vi "formatMsgDetails.vi"(8 "error in (no error)":errorcluster, 9 "msgTypeEnum":T1, 10 "msgCluster":T2={"msgName"="move", "msgDetails"=""}, 11 "TcpServer.lvclass":refnum<class "TcpServer.lvclass">) -> (0 "error out":errorcluster, 2 "jsonString":string, 3 "TcpServer.lvclass":refnum<class "TcpServer.lvclass">)   [LabVIEW 2018, in "TcpServer.lvclass"]
doc: "Convert the event or the telemetry message into a JSON format. You can choose if is event or telemetry with the message type enum provided. If msgName has an empty string, an error message will be created to inform other processes about this error."
uses:
  TcpServer.lvclass
  typedef/msgTypeDef.ctl
  typedef/msgTypeEnum.ctl
  <vilib>/Utility/error.llb/Error Cluster From Error Code.vi
  <vilib>/ErrorRing/Error Ring.xnode
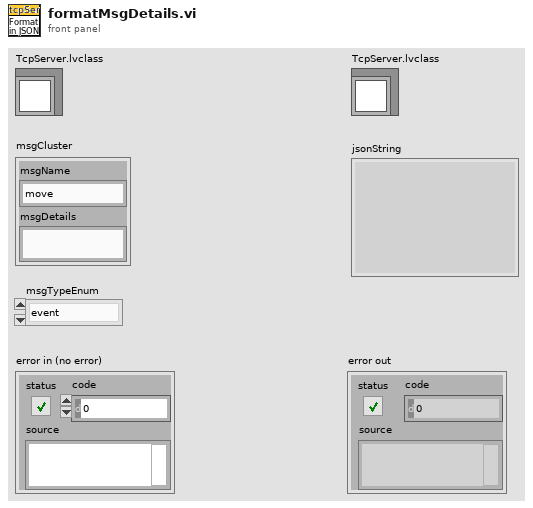
[diagram p1: front panel]
types:
  T1 = typedef "TcpServer.lvclass/msgTypeEnum.ctl" = enum16{"event", "telemetry"}
  T2 = typedef "TcpServer.lvclass/msgTypeDef.ctl" = cluster{"msgName":string, "msgDetails":string}
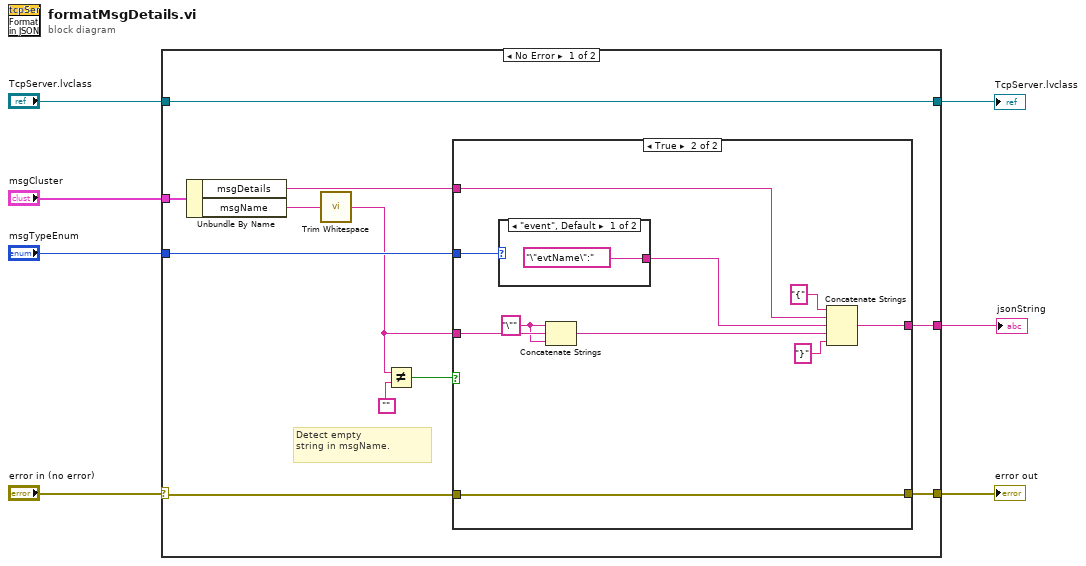
[diagram p0: block diagram]
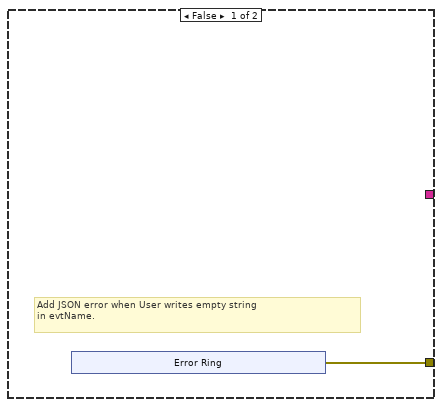
[diagram p2: hidden frame]
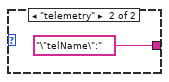
[diagram p3: hidden frame]
diagram:
  n1 = case shown="No Error" "error in (no error)" {
    selector: "error in (no error)" -> [w14 w36]
    tunnel: [w18 _] -> w3
    tunnel: "TcpServer.lvclass" -> [w17 w37]
    tunnel: [w17 w37] -> w5
    tunnel: [w13 w36] -> w4
    tunnel: "msgTypeEnum" -> [w12 _]
    tunnel: "msgCluster" -> [w10 _]
    frame No Error {
      # "Detect empty\nstring in msgName."
      n2 = Unbundle By Name(w10) -> ("msgDetails"=w8:string, "msgName"=w9:string)
      n3 = call <vilib>:"Trim Whitespace.vi"("string"=w9) -> ("trimmed string"=w11:string)  [unwired: 1 in]
      n4 = Not Equal?(x=w11, y="") -> (x != y?=w15:bool)
      n5 = case shown="True" w15 {
        tunnel: [_ w33] -> w18
        tunnel: w8 -> [_ w26]
        tunnel: w11 -> [_ w32]
        tunnel: w14 -> [_ w28]
        tunnel: [w19 w28] -> w13
        tunnel: w12 -> [_ w27]
        frame False {
          # "Add JSON error when User writes empty string\nin evtName."
          n6 = xnode "Error Ring"() -> ("error out"=w19:errorcluster)
        }
        frame True {
          w29 = "\"" ("string")
          n7 = case shown="\"event\", Default" w27 {
            tunnel: ["\"evtName\":" "\"telName\":"] -> w25
            frame "event", Default {
            }
            frame "telemetry" {
            }
          }
          n8 = Concatenate Strings(w29, w32, w29) -> (w24:string)
          n9 = Concatenate Strings("{" ("string"), w26, w25, w24, "}" ("string")) -> (w33:string)
        }
      }
    }
    frame Error {
    }
  }
  "jsonString" <- w3
  "error out" <- w4
  "TcpServer.lvclass" <- w5
